vi "escapeXML.vi"(10 "Input String":string) -> (2 "XML-escaped String":string)   [LabVIEW 2013, in "Caraya.lvlib" / "Test Report.JUnit.lvclass"]
uses:
  Test Report.JUnit.lvclass
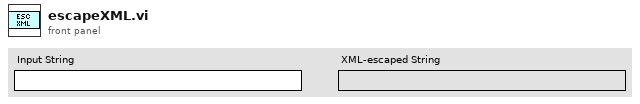
[diagram p1: front panel]
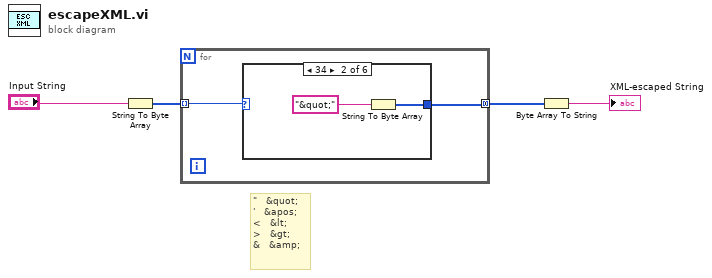
[diagram p0: block diagram]
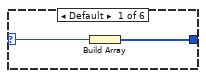
[diagram p2: hidden frame]
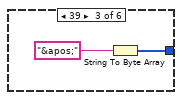
[diagram p3: hidden frame]
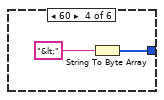
[diagram p4: hidden frame]
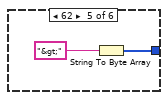
[diagram p5: hidden frame]
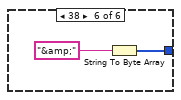
[diagram p6: hidden frame]
diagram:
  # "\"   &quot;\n'   &apos;\n<   &lt;\n>   &gt;\n&   &amp;"
  n1 = String To Byte Array(string="Input String") -> (unsigned byte array=w3:u8[])
  n2 = for {
    tunnel: w3 -> [w6] mode=indexing
    tunnel: [w5] -> w1 mode=concatenating
    n3 = case shown="34" w6 {
      selector: w6 -> [w8 _ _ _ _ _]
      tunnel: [w7 w10 w12 w14 w16 w18] -> w5
      frame Default {
        n4 = Build Array(w8) -> (w7:u8[])
      }
      frame 34 {
        n5 = String To Byte Array(string="&quot;" ("Input String")) -> (unsigned byte array=w10:u8[])
      }
      frame 39 {
        n6 = String To Byte Array(string="&apos;" ("Input String")) -> (unsigned byte array=w12:u8[])
      }
      frame 60 {
        n7 = String To Byte Array(string="&lt;" ("Input String")) -> (unsigned byte array=w14:u8[])
      }
      frame 62 {
        n8 = String To Byte Array(string="&gt;" ("Input String")) -> (unsigned byte array=w16:u8[])
      }
      frame 38 {
        n9 = String To Byte Array(string="&amp;" ("Input String")) -> (unsigned byte array=w18:u8[])
      }
    }
  }
  n10 = Byte Array To String(unsigned byte array=w1) -> (string=→"XML-escaped String":string)
